vi "Temp.vi"(11 "string":string) -> ()   [LabVIEW 2018]
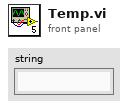
[diagram p1: front panel]
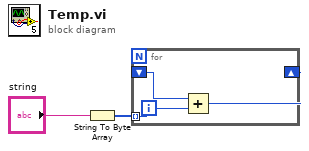
[diagram p0: block diagram]
diagram:
  n1 = String To Byte Array(string="string") -> (unsigned byte array=w1:u8[])
  n2 = for {
    shift-right: [w4] -> _
    shift-left: _ -> [w5]
    tunnel: w1 -> [w3] mode=indexing
    n3 = Add(x=w5, y=w3) -> (x+y=w4:u8)
  }
